vi "Untitled 1 (SubVI).vi"(0 "Numeric 10":dbl, 1 "Numeric 11":dbl, 2 "Numeric 6":dbl, 3 "P0":dbl=0.5, 4 "r":dbl=1.0, 5 "q":dbl=1.0, 6 "Numeric 5":dbl, 8 "Numeric 9":dbl, 10 "Particle Reports (Pixels)":T1(array[cluster])) -> (12 "Left":dbl, 13 "Bounding Rect.Right":dbl, 14 "Right":bool, 15 "Bounding Rect.Left":dbl, 16 "Numeric 7":dbl, 17 "left Angle":dbl, 18 "Numeric 4":dbl, 19 "right Angle":dbl, 20 "Numeric 3":dbl, 21 "Average Cam Distance":dbl, 22 "Right 2":dbl, 23 "Numeric 8":dbl, 24 "Numeric 2":dbl, 25 "Numeric":dbl, 26 "Average Cam Angle":dbl)   [LabVIEW 2016]
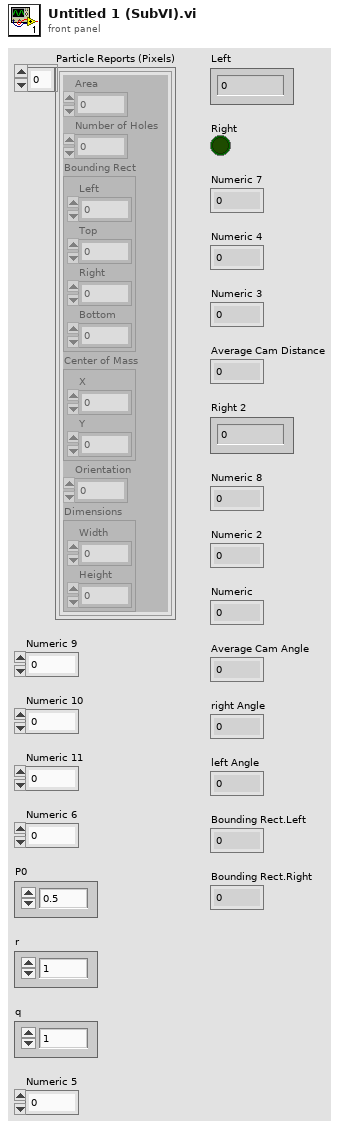
[diagram p1: front panel]
types:
  T1 = cluster{"Area":dbl, "Number of Holes":dbl, "Bounding Rect":cluster{"Left":dbl, "Top":dbl, "Right":dbl, "Bottom":dbl}, "Center of Mass":cluster{"X":dbl, "Y":dbl}, "Orientation":dbl, "Dimensions":cluster{"Width":dbl, "Height":dbl}}[]
  T2 = cluster{"Area":dbl, "Number of Holes":dbl, "Bounding Rect":cluster{"Left":dbl, "Top":dbl, "Right":dbl, "Bottom":dbl}, "Center of Mass":cluster{"X":dbl, "Y":dbl}, "Orientation":dbl, "Dimensions":cluster{"Width":dbl, "Height":dbl}}
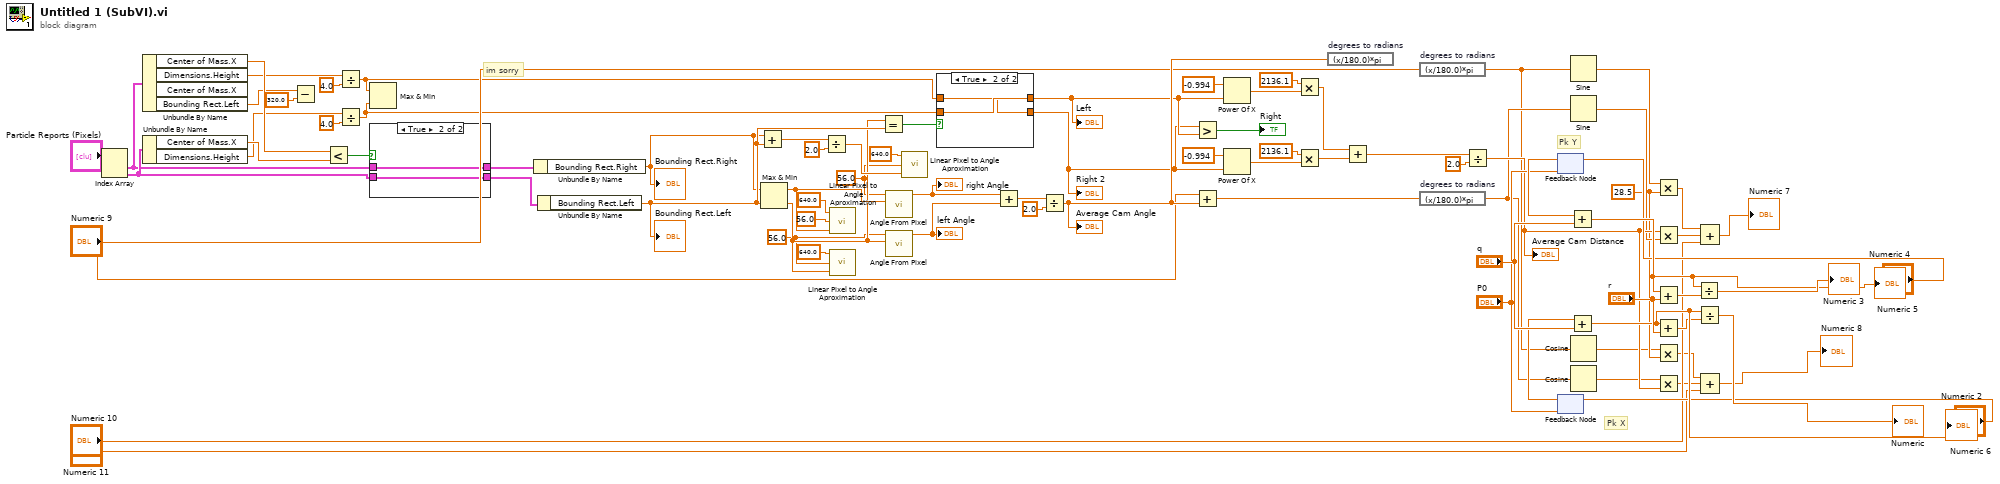
[diagram p0: block diagram]
diagram:
  w38 = 28.5 ("y")
  w48 = 56.0 ("Axis Fov")
  w47 = 56.0 ("Axis Fov")
  # "Pk Y"
  # "Pk X"
  # "im sorry"
  n1 = Index Array(array="Particle Reports (Pixels)") -> (element #1=w56:T2, element #2=w57:T2)  [unwired: 2 in]
  n2 = Unbundle By Name(w56) -> ("Center of Mass.X"=w54:dbl, "Dimensions.Height"=w13:dbl, "Bounding Rect.Left"=w25:dbl)  [unwired: 1 out]
  n3 = Unbundle By Name(w57) -> ("Center of Mass.X"=w61:dbl, "Dimensions.Height"=w15:dbl)
  n4 = Subtract(x=w25, y=320.0) -> ()  [unwired: 1 out]
  n5 = Less?(x=w54, y=w61) -> (x < y?=w55:bool)
  n6 = Divide(x=w13, y=4.0) -> (x/y=w12:dbl)
  n7 = Divide(x=w15, y=4.0) -> (x/y=w16:dbl)
  n8 = Max & Min(x=w12, y=w16) -> ()  [unwired: 2 out]
  n9 = case shown="True" w55 {
    tunnel: w56 -> [w80 w83]
    tunnel: [w81 w83] -> w58
    tunnel: w57 -> [w81 w82]
    tunnel: [w80 w82] -> w59
    frame False {
    }
    frame True {
    }
  }
  n10 = Unbundle By Name(w58) -> ("Bounding Rect.Right"=w60:dbl)
  "Bounding Rect.Right" <- w60
  n11 = Unbundle By Name(w59) -> ("Bounding Rect.Left"=w62:dbl)
  "Bounding Rect.Left" <- w62
  n12 = Add(x=w60, y=w62) -> (x+y=w1:dbl)
  n13 = Max & Min(x=w60, y=w62) -> (max(x,y)=w52:dbl, min(x,y)=w49:dbl)
  n14 = Divide(x=w1, y=2.0) -> (x/y=w51:dbl)
  n15 = call "Linear Pixel to Angle Aproximation.vi"("Axis Pixel"=w52, "Axis Fov"=56.0, "Axis Lengh"=640.0) -> ()  [unwired: 1 out]
  n16 = call "Linear Pixel to Angle Aproximation.vi"("Axis Pixel"=w49, "Axis Fov"=w48, "Axis Lengh"=640.0) -> ()  [unwired: 1 out]
  n17 = Equal?(x=w49, y=w62) -> (x = y?=w6:bool)
  n18 = call "Angle From Pixel.vi"("Pixel"=w52, "Angle Aperture"=w47) -> ("Theta"=w53:dbl)  [unwired: 9 in]
  "right Angle" <- w53
  n19 = call "Angle From Pixel.vi"("Pixel"=w49, "Angle Aperture"=w48) -> ("Theta"=w50:dbl)  [unwired: 9 in]
  "left Angle" <- w50
  n20 = call "Linear Pixel to Angle Aproximation.vi"("Axis Pixel"=w51, "Axis Fov"=w47, "Axis Lengh"=640.0) -> ()  [unwired: 1 out]
  n21 = case shown="True" w6 {
    tunnel: w16 -> [w84 w87]
    tunnel: [w85 w87] -> w22
    tunnel: w12 -> [w85 w86]
    tunnel: [w84 w86] -> w18
    frame False {
    }
    frame True {
    }
  }
  "Left" <- w22
  "Right 2" <- w18
  n22 = Add(x=w53, y=w50) -> (x+y=w30:dbl)
  n23 = Divide(x=w30, y=2.0) -> (x/y=w63:dbl)
  "Average Cam Angle" <- w63
  n24 = Greater?(x=w18, y=w22) -> (0:→"Right":bool)
  n25 = Add(x="Numeric 9", y=w63) -> (x+y=w45:dbl)
  n26 = Power Of X(1:w22, 2:-0.994 ("x")) -> (0:w21:dbl)
  n27 = Power Of X(1:w18, 2:-0.994 ("x")) -> (0:w3:dbl)
  n28 = Multiply(x=2136.1, y=w21) -> (x*y=w26:dbl)
  n29 = Multiply(x=2136.1, y=w3) -> (x*y=w31:dbl)
  n30 = expression code="(x/180.0)*pi" "degrees to radians"(w63) -> ()  [unwired: 1 out]
  n31 = Add(x=w26, y=w31) -> (x+y=w27:dbl)
  n32 = expression code="(x/180.0)*pi" "degrees to radians"("Numeric 9") -> (w42:dbl)
  n33 = expression code="(x/180.0)*pi" "degrees to radians"(w45) -> (w46:dbl)
  n34 = Divide(x=w27, y=2.0) -> (x/y=w64:dbl)
  "Average Cam Distance" <- w64
  n35 = feedback #1("P0") -> (w70:dbl)
  n36 = feedback-in #1("Numeric 5") -> ()
  n37 = feedback #2("P0") -> (w67:dbl)
  n38 = feedback-in #2("Numeric 6") -> ()
  n39 = Add(x=w70, y="q") -> (x+y=w73:dbl)
  "Numeric 4" <- w73
  n40 = Add(x=w67, y="q") -> (x+y=w77:dbl)
  "Numeric 2" <- w77
  n41 = Sine(x=w42) -> (sin(x)=w37:dbl)
  n42 = Sine(x=w46) -> (sin(x)=w39:dbl)
  n43 = Cosine(x=w42) -> (cos(x)=w32:dbl)
  n44 = Cosine(x=w46) -> (cos(x)=w35:dbl)
  n45 = Multiply(x=w37, y=w38) -> (x*y=w36:dbl)
  n46 = Multiply(x=w64, y=w39) -> (x*y=w43:dbl)
  n47 = Add(x=w73, y="r") -> (x+y=w74:dbl)
  n48 = Add(x=w77, y="r") -> (x+y=w76:dbl)
  n49 = Multiply(x=w32, y=w38) -> (x*y=w33:dbl)
  n50 = Multiply(x=w35, y=w64) -> (x*y=w34:dbl)
  n51 = Divide(x=w73, y=w74) -> (x/y=→"Numeric 3":dbl)
  n52 = Divide(x=w77, y=w76) -> (x/y=→"Numeric":dbl)
  n53 = Compound Arithmetic op=ADD(w36, w43, "Numeric 10") -> (→"Numeric 7":dbl)
  n54 = Compound Arithmetic op=ADD(w33, w34, "Numeric 11") -> (→"Numeric 8":dbl)
